vi "ReadWebsocketPacketHeader.vi"(8 "error in":errorcluster, 11 "connection ID":refnum<k5>) -> (0 "error out":errorcluster, 1 "final":bool, 2 "payload length":u64, 3 "connection ID out":refnum<k5>, 4 "mask value":u32 format="%.0x", 5 "opcode":T1, 6 "mask":bool)   [LabVIEW 2014, in "Raspberry Pi Compatible Compiler for LabVIEW.lvlib" / "Websocket.lvlib"]
uses:
  Websocket.lvlib
  WebsocketFrameTypes_TD.ctl
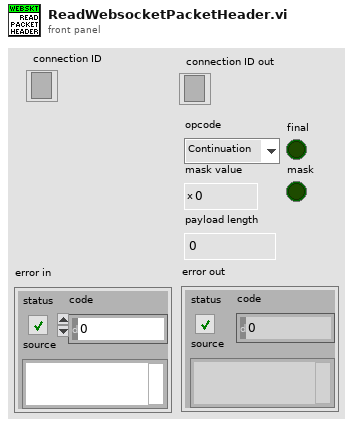
[diagram p1: front panel]
types:
  T1 = typedef "Raspberry Pi Compatible Compiler for LabVIEW.lvlib/Websocket.lvlib/WebsocketFrameTypes_TD.ctl" = enum8{"Continuation", "Text", "Binary", "Reserved 1", "Reserved 2", "Reserved 3", "Reserved 4", "Reserved 5", "Close", "Ping", "Pong", "Reserved 6", "Reserved 7", "Reserved 8", "Reserved 9", "Reserved 10"}
  T2 = enum16{"big-endian, network order", "native, host order", "little-endian"}
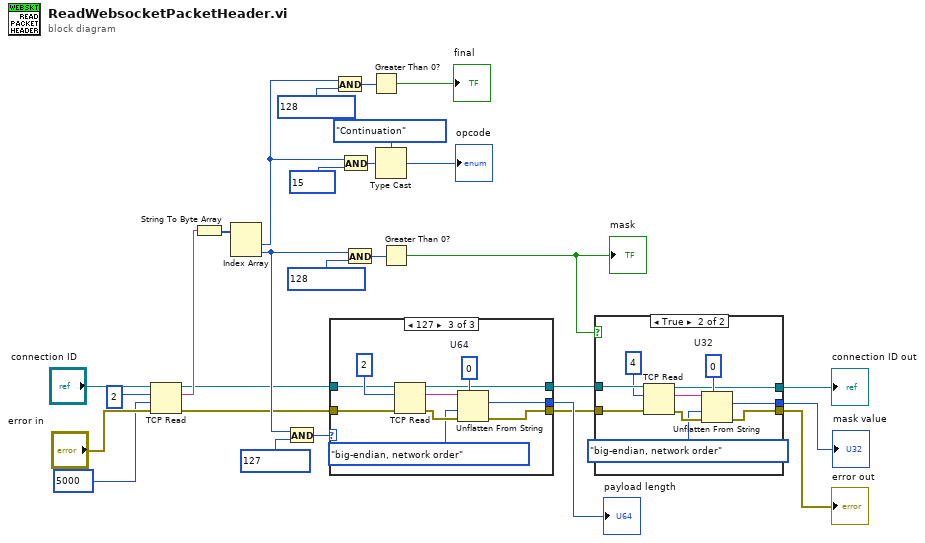
[diagram p0: block diagram]
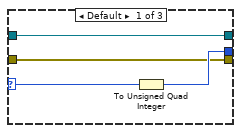
[diagram p3: hidden frame]
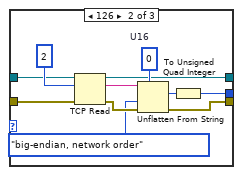
[diagram p4: hidden frame]
diagram:
  n1 = TCP Read(connection ID="connection ID", bytes to read=2, error in (no error)="error in", 9:5000 ("timeout ms (25000)")) -> (connection ID out=w10:refnum<k5>, data out=w27:string, error out=w9:errorcluster)  [unwired: 1 in]
  n2 = String To Byte Array(string=w27) -> (unsigned byte array=w26:u8[])
  n3 = Index Array(array=w26) -> (element #1=w19:u8, element #2=w12:u8)  [unwired: 2 in]
  n4 = And(x=w12, y=u8 127) -> (x .and. y?=w11:u8)
  n5 = case shown="127" w11 {
    selector: w11 -> [w32 _ _]
    tunnel: [w31 w35 w44] -> w8
    tunnel: w10 -> [w29 w42 w52]
    tunnel: w9 -> [w30 w41 w51]
    tunnel: [w29 w34 w46] -> w7
    tunnel: [w30 w33 w45] -> w6
    frame Default {
      n6 = To Unsigned Quad Integer(1:w32) -> (0:w31:u64)
    }
    frame 126 {
      w37 = u16 0  # U16
      n7 = TCP Read(connection ID=w42, bytes to read=2, error in (no error)=w41) -> (connection ID out=w34:refnum<k5>, data out=w40:string, error out=w39:errorcluster)  [unwired: 2 in]
      n8 = Unflatten From String(type=w37, binary string=w40, byte order (0:big-endian, network order)=T2."big-endian, network order", error in (no error)=w39) -> (value=w36:u16, error out=w33:errorcluster)  [unwired: 1 in, 1 out]
      n9 = To Unsigned Quad Integer(1:w36) -> (0:w35:u64)
    }
    frame 127 {
      w47 = u64 0  # U64
      n10 = TCP Read(connection ID=w52, bytes to read=2, error in (no error)=w51) -> (connection ID out=w46:refnum<k5>, data out=w50:string, error out=w49:errorcluster)  [unwired: 2 in]
      n11 = Unflatten From String(type=w47, binary string=w50, byte order (0:big-endian, network order)=T2."big-endian, network order", error in (no error)=w49) -> (value=w44:u64, error out=w45:errorcluster)  [unwired: 1 in, 1 out]
    }
  }
  "payload length" <- w8
  n12 = And(x=w19, y=u8 128) -> (x .and. y?=w23:u8)
  n13 = And(x=w19, y=u8 15) -> (x .and. y?=w17:u8)
  n14 = And(x=w12, y=u8 128) -> (x .and. y?=w14:u8)
  n15 = Greater Than 0?(x=w23) -> (x > 0?=→"final":bool)
  n16 = Type Cast(type=WebsocketFrameTypes_TD."Continuation", x=w17) -> (*(type *) &x=→"opcode":T1)
  n17 = Greater Than 0?(x=w14) -> (x > 0?=w5:bool)
  "mask" <- w5
  n18 = case shown="True" w5 {
    tunnel: w7 -> [w55 w64]
    tunnel: w6 -> [w54 w65]
    tunnel: [_ w58] -> w2
    tunnel: [w55 w57] -> w4
    tunnel: [w54 w56] -> w3
    frame False {
    }
    frame True {
      w59 = u32 0  # U32
      n19 = TCP Read(connection ID=w64, bytes to read=4, error in (no error)=w65) -> (connection ID out=w57:refnum<k5>, data out=w61:string, error out=w62:errorcluster)  [unwired: 2 in]
      n20 = Unflatten From String(type=w59, binary string=w61, byte order (0:big-endian, network order)=T2."big-endian, network order", error in (no error)=w62) -> (value=w58:u32, error out=w56:errorcluster)  [unwired: 1 in, 1 out]
    }
  }
  "error out" <- w3
  "connection ID out" <- w4
  "mask value" <- w2
